vi "PQ_asynchron_sample.vi"() -> ()   [LabVIEW 2019, in "libpqutility.lvlib"]
doc: "example to show how to communicate asyncronous wir PostgreSQL"
uses:
  libpqutility.lvlib
  libpqlv/libpqlv.lvlib
panel:
  out "parameterstatus":string
  out "PQbinaryTuples":i32
  out "PQprotocolVersion":u32
  out "PQnTuples":i32
  out "PQsendQuery":i32
  out "PQerrorMessage":string
  out "PQresultErrorMessage":string
  in  "query":string
  out "PQresultStatus":T1(ring)
  out "PQStatus":T2(ring)
  out "Tabelle":string[][](table)
  in  "conninfo":string
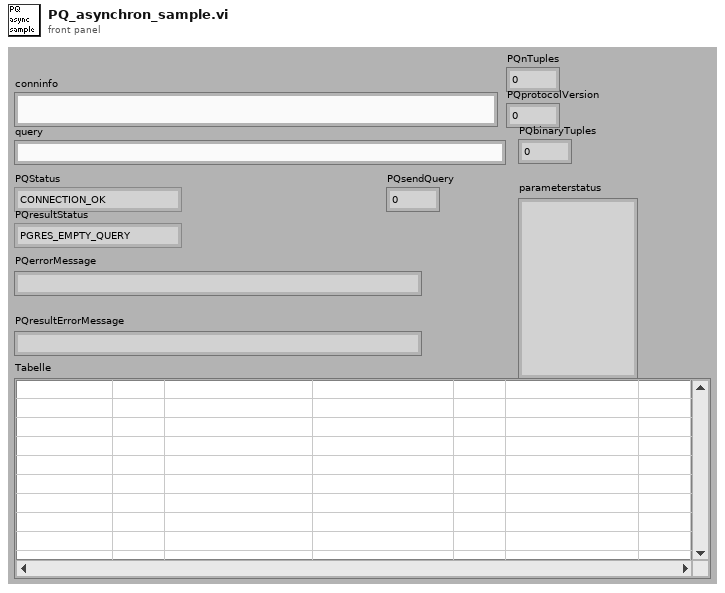
[diagram p1: front panel]
types:
  T1 = enum16{"PGRES_EMPTY_QUERY", "PGRES_COMMAND_OK", "PGRES_TUPLES_OK", "PGRES_COPY_OUT", "PGRES_COPY_IN", "PGRES_BAD_RESPONSE", "PGRES_NONFATAL_ERROR", "PGRES_FATAL_ERROR"}
  T2 = enum16{"CONNECTION_OK", "CONNECTION_BAD", "CONNECTION_STARTED", "CONNECTION_MADE", "CONNECTION_AWAITING_RESPONSE", "CONNECTION_AUTH_OK", "CONNECTION_SETENV", "CONNECTION_SSL_STARTUP", "CONNECTION_NEEDED"}
  T3 = enum32{"CONNECTION_OK", "CONNECTION_BAD", "CONNECTION_STARTED", "CONNECTION_MADE", "CONNECTION_AWAITING_RESPONSE", "CONNECTION_AUTH_OK", "CONNECTION_SETENV", "CONNECTION_SSL_STARTUP", "CONNECTION_NEEDED"}
  T4 = enum32{"PGRES_EMPTY_QUERY", "PGRES_COMMAND_OK", "PGRES_TUPLES_OK", "PGRES_COPY_OUT", "PGRES_COPY_IN", "PGRES_BAD_RESPONSE", "PGRES_NONFATAL_ERROR", "PGRES_FATAL_ERROR"}
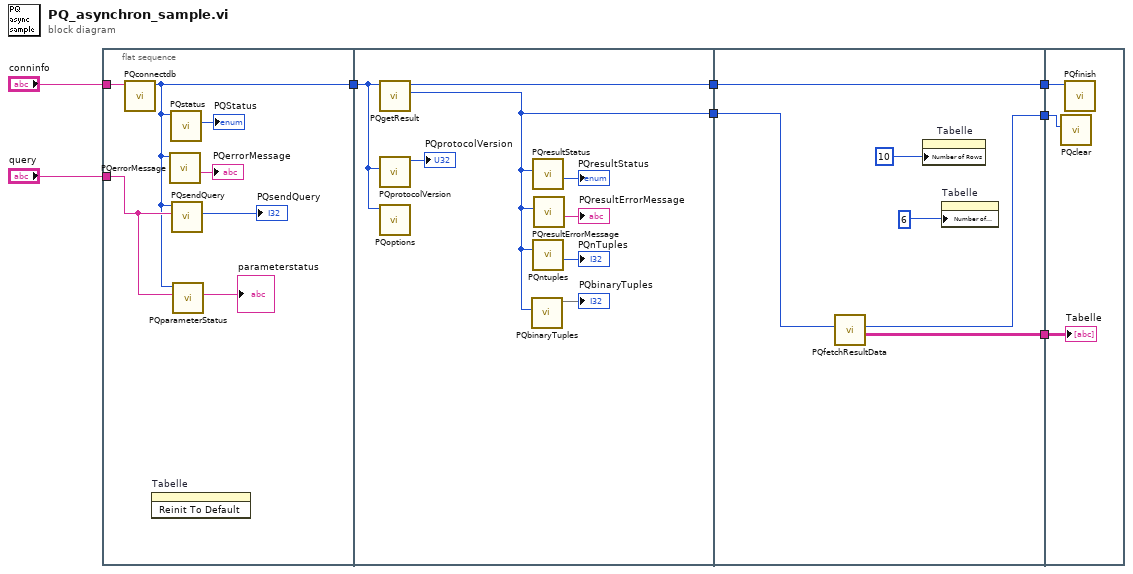
[diagram p0: block diagram]
diagram:
  n1 = flat-sequence {
    tunnel: "conninfo" -> [w15]
    tunnel: "query" -> [w11]
    tunnel: [w10] -> w2
    tunnel: [w16] -> w5
    tunnel: [w20] -> w3
    tunnel: w2 -> [w21]
    tunnel: [w27] -> w6
    tunnel: w5 -> [w27]
    tunnel: [w25] -> w4
    tunnel: w3 -> [w26]
    tunnel: [w24] -> w1
    tunnel: w6 -> [w30]
    tunnel: w4 -> [w32]
    tunnel: w1 -> [w31]
    frame #0 {
      n2 = call "PQconnectdb.vi"("conninfo"=w15) -> ("conn"=w10:u32)  [unwired: 9 in, 1 out]
      n3 = invoke on="Tabelle" class="Tbl (strikt)" method="Reinit To Default"() -> ()  [unwired: 3 in, 3 out]
      n4 = call "PQerrorMessage.vi"("conn"=w10) -> ("PQerrorMessage"=→"PQerrorMessage":string)  [unwired: 8 in, 2 out]
      n5 = call "PQstatus.vi"("conn"=w10) -> ("PQStatus"=→"PQStatus":T3)  [unwired: 8 in, 2 out]
      n6 = call "PQsendQuery.vi"("query"=w11, "conn"=w10) -> ("PQsendQuery"=→"PQsendQuery":i32)  [unwired: 7 in, 2 out]
      n7 = call "PQparameterStatus.vi"("paramName"=w11, "conn"=w10) -> ("parameterstatus"=→"parameterstatus":string)  [unwired: 6 in, 2 out]
    }
    frame #1 {
      n8 = call "PQgetResult.vi"("conn"=w21) -> ("PGresult"=w20:u32, "conn_out"=w16:u32)  [unwired: 8 in, 1 out]
      n9 = call "PQprotocolVersion.vi"("conn"=w21) -> ("PQprotocolVersion"=→"PQprotocolVersion":u32)  [unwired: 9 in, 1 out]
      n10 = call "PQoptions.vi"("conn"=w21) -> ()  [unwired: 7 in, 3 out]
      n11 = call "PQbinaryTuples.vi"("res"=w20) -> (3:→"PQbinaryTuples")  [unwired: 7 in, 3 out]
      n12 = call "PQresultStatus.vi"("res"=w20) -> ("PQresultStatus"=→"PQresultStatus":T4)  [unwired: 8 in, 2 out]
      n13 = call "PQntuples.vi"("res"=w20) -> ("PQnTuples"=→"PQnTuples":i32)  [unwired: 8 in, 2 out]
      n14 = call "PQresultErrorMessage.vi"("res"=w20) -> ("PQresultErrorMessage"=→"PQresultErrorMessage":string)  [unwired: 8 in, 2 out]
    }
    frame #2 {
      n15 = call "PQfetchResultData.vi"("res"=w26) -> ("Data"=w24:string[][], "res_out"=w25:u32)  [unwired: 5 in, 4 out]
      n16 = property on="Tabelle" class="Tbl (strict)"("Number of Rows"=u32 10 ("Zeilenanzahl")) -> ()  [unwired: 2 in, 2 out]
      n17 = property on="Tabelle" class="Tbl (strict)"("Number of Columns"=u32 6 ("Spaltenanzahl")) -> ()  [unwired: 2 in, 2 out]
    }
    frame #3 {
      n18 = call "PQclear.vi"("res"=w32) -> ()  [unwired: 9 in, 2 out]
      n19 = call "PQfinish.vi"("conn"=w30) -> ()  [unwired: 10 in, 1 out]
      "Tabelle" <- w31
    }
  }
